vi "Take and analyse picture.vi"(0 "Training image on/off":bool, 1 "8 Insects or less":bool, 2 "Session Out in":T3, 3 "Refnum in":T1, 5 "error in (no error)":errorcluster, 6 "Sample ID":string, 8 "Safe pictures":bool) -> (9 "error out":errorcluster, 10 "output cluster":T2, 14 "Insect-data-array (out of range removed)":dbl[][](array[numeric]), 16 "Number of objects":i32, 17 "Session Out out":T3, 18 "Tegne cirkel array":dbl[][](array[numeric]), 19 "Black image error":bool)   [LabVIEW 2024]
doc: "Collects an image and runs it throu the vision asistent. Then transforms output data to sutible outlets and formats."
uses:
  <vilib>/userDefined/High Color/IMAQdx.ctl
  <vilib>/vision/Image Controls.llb/IMAQ Image.ctl
  <vilib>/vision/NI_Vision_Development_Module.lvlib
  <vilib>/vision/driver/NI_Vision_Acquisition_Software.lvlib
panel:
  out "Camera feed":T1(plugin-control)
  in  "Boolean":bool
  out "Image from vision assistant 2":T1(plugin-control)
  out "T_and_A Stoped":bool
  out "Match Score (Color Matching 1)":i32[](array[numeric])
  out "Objects after sorting":string[][](array[string])
  out "Image from vision assistant":T1(plugin-control)
  in  "Stop program":bool
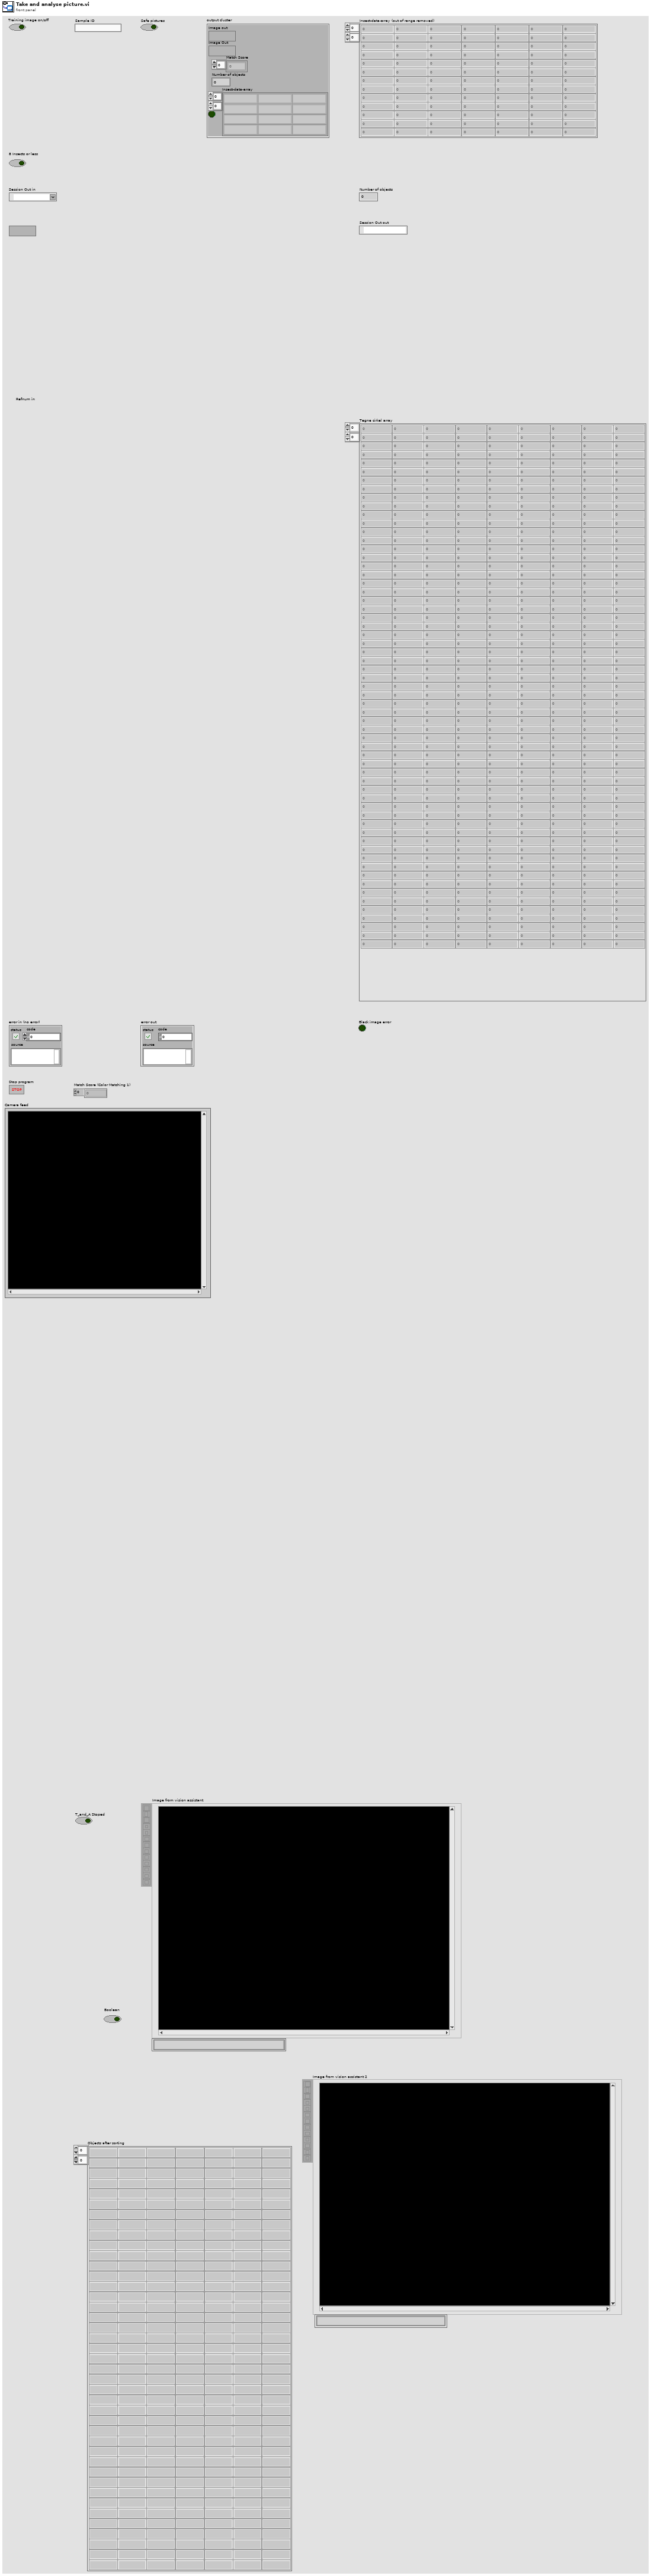
[diagram p1: front panel]
types:
  T1 = typedef "IMAQ Image.ctl" = refnum<image>
  T2 = cluster{"Image out":T1, "Image Out":T1, "Match Score":i32[], "Number of objects":i32, "Insect-data-array":string[][], bool}
  T3 = typedef "IMAQdx.ctl" = refnum<k21>
  T4 = cluster{"Measurement Parameter":i32, "Range Lower Value":dbl, "Range Upper Value":dbl, "Range":bool, "Measurement Type":bool}[]
  T5 = cluster{"Image out":T1, "Image Out":T1, "Match Score (Color Matching 1)":i32[], "Number of objects":i32, "Insect-data-array":string[][], bool}
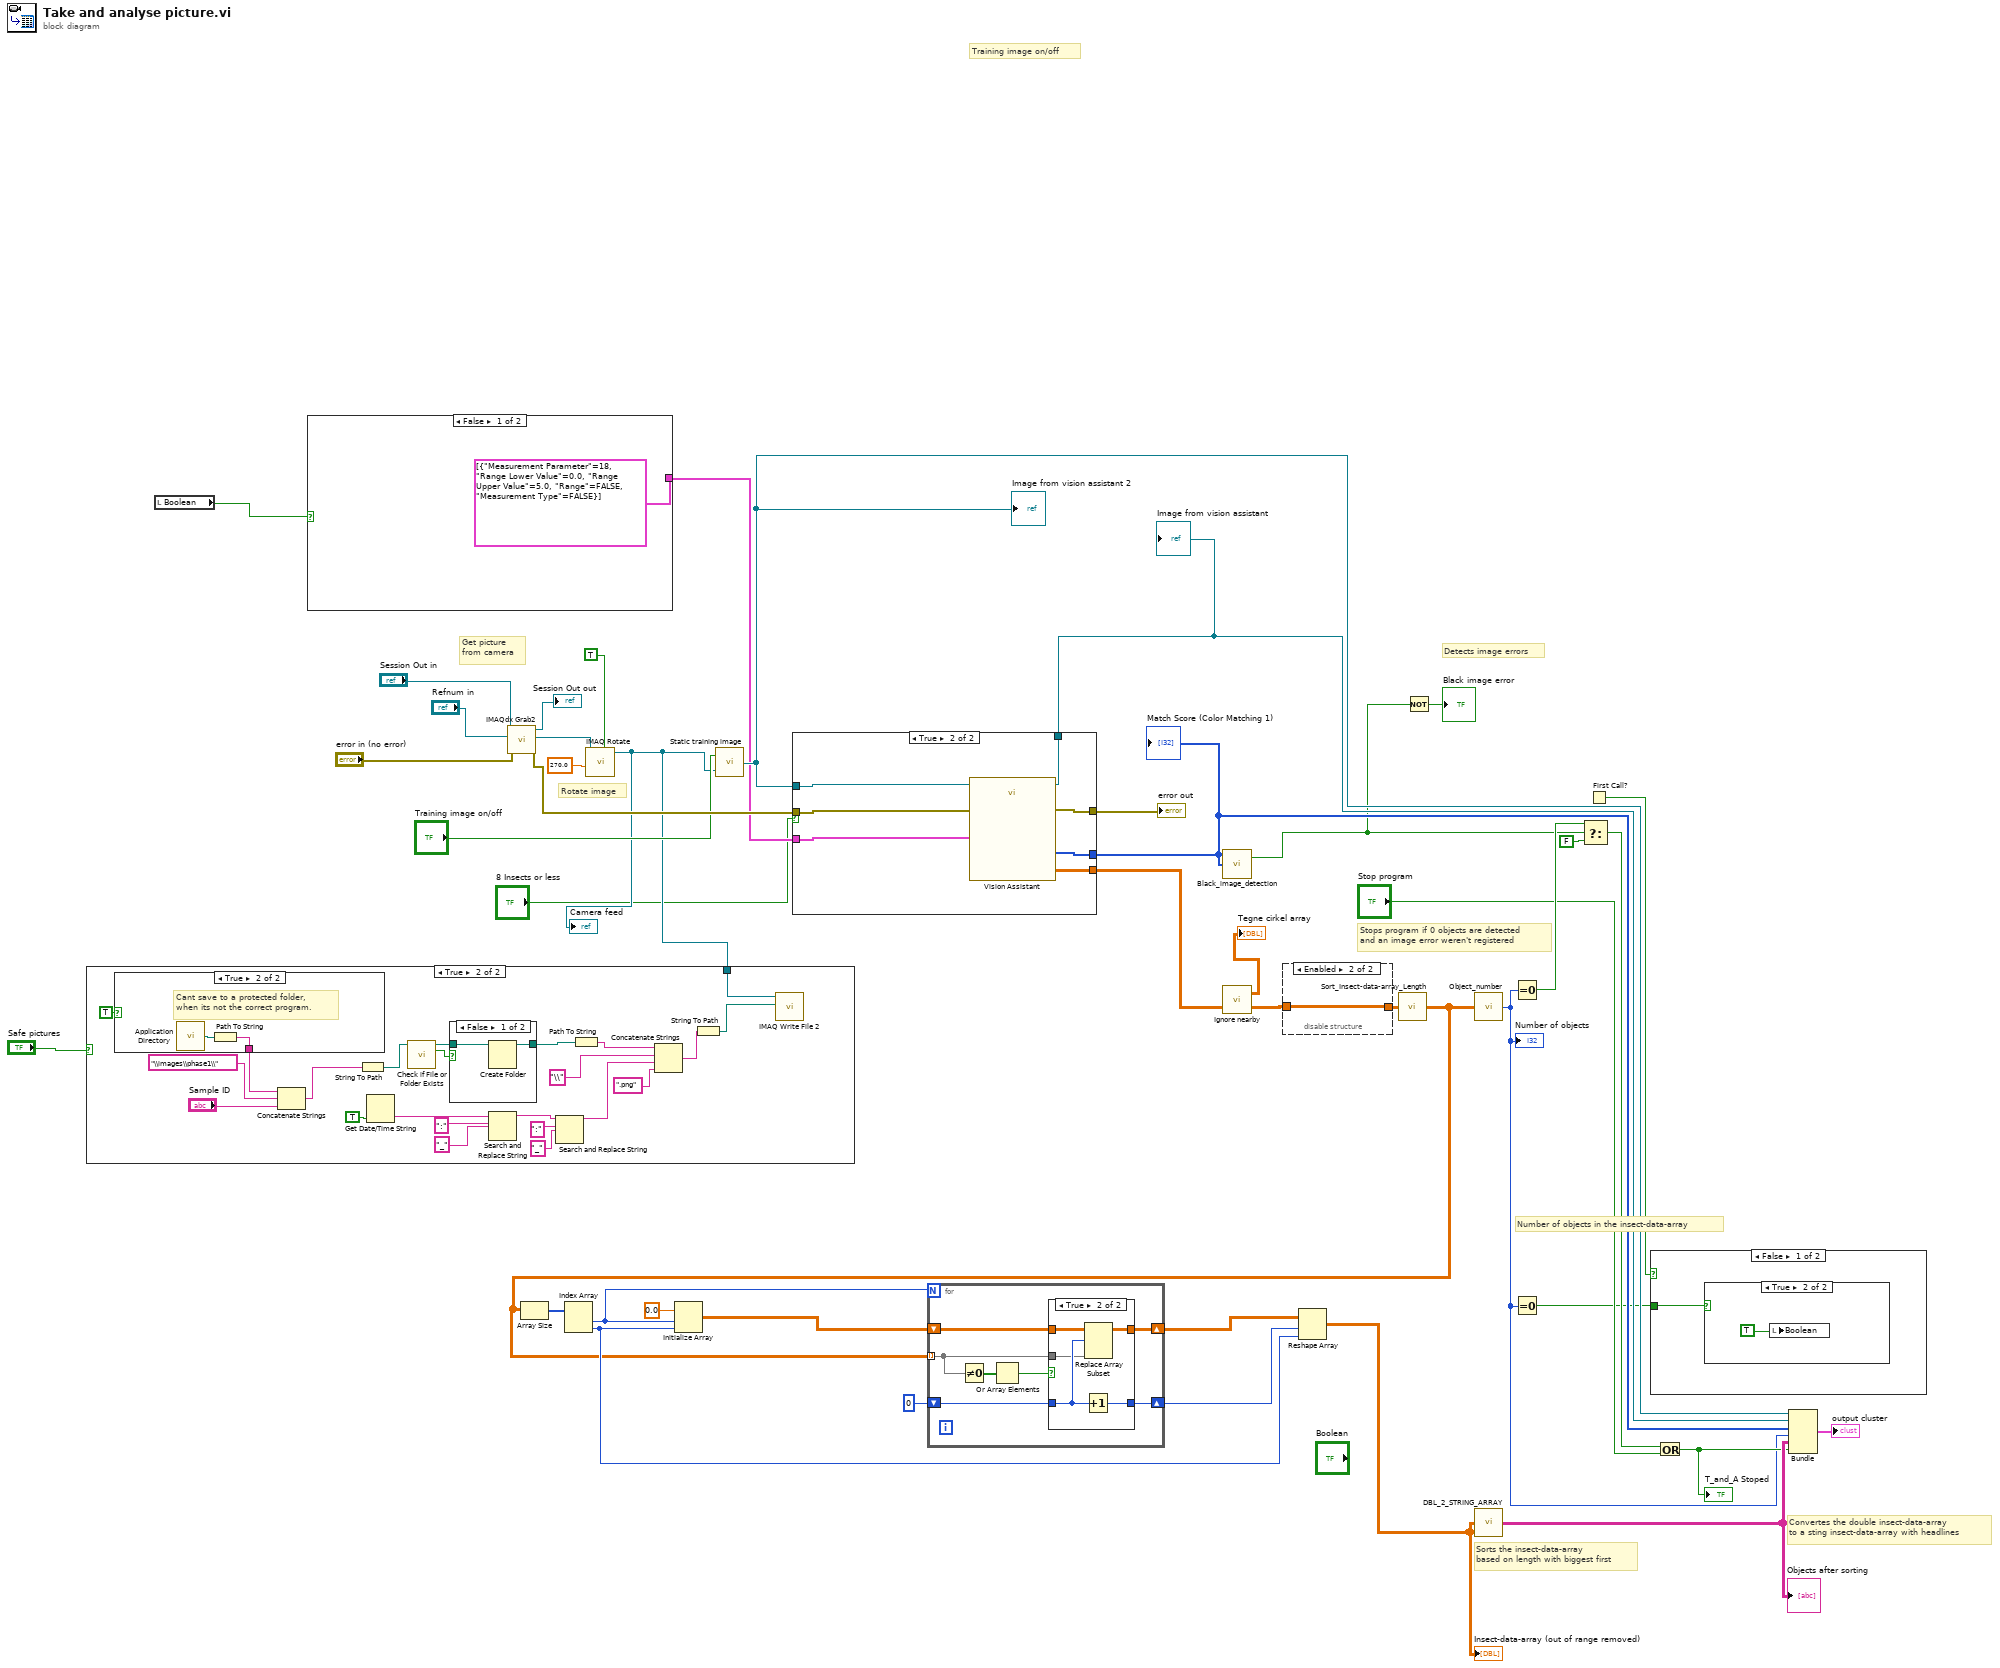
[diagram p0: block diagram]
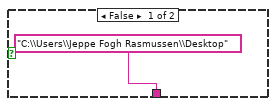
[diagram p3: hidden frame]
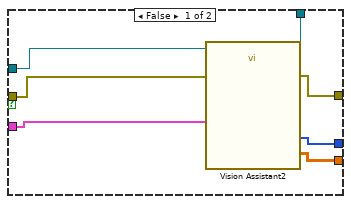
[diagram p5: hidden frame]
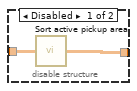
[diagram p6: hidden frame]
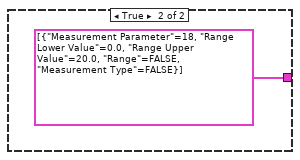
[diagram p8: hidden frame]
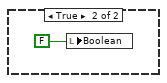
[diagram p10: hidden frame]
diagram:
  # "Detects image errors"
  # "Stops program if 0 objects are detected \nand an image error weren't registered"
  # "Number of objects in the insect-data-array"
  # "Convertes the double insect-data-array\nto a sting insect-data-array with headlines"
  # "Get picture \nfrom camera"
  # "Rotate image"
  # "Training image on/off"
  # "Sorts the insect-data-array\nbased on length with biggest first"
  n1 = local read "Boolean"() -> (w22:bool)
  n2 = case shown="False" w22 {
    tunnel: [T4 [{"Measurement Parameter"=18, "Range Lower Value"=0.0, "Range Upper Value"=5.0, "Range"=FALSE, "Measurement Type"=FALSE}] ("Selection Values (Particle Filter 2)") T4 [{"Measurement Parameter"=18, "Range Lower Value"=0.0, "Range Upper Value"=20.0, "Range"=FALSE, "Measurement Type"=FALSE}] ("Selection Values (Particle Filter 2)")] -> w24
    frame False {
    }
    frame True {
    }
  }
  n3 = call <vilib>:"IMAQdx Grab2.vi"("error in"="error in (no error)", "Image In"="Refnum in", "Session In"="Session Out in") -> ("error out"=w34:errorcluster, "Image Out"=w40:T1, "Session Out"=→"Session Out out":T3)  [unwired: 5 in, 1 out]
  n4 = call "IMAQ Rotate"("Maintain Size"=TRUE, "Angle (degrees)"=sgl 270.0, "Image Src"=w40) -> ("Image Dst Out"=w5:T1)  [unwired: 7 in, 1 out]
  "Camera feed" <- w5
  n5 = case shown="True" "Safe pictures" {
    tunnel: w5 -> [_ w69]
    frame False {
    }
    frame True {
      n6 = case shown="True" TRUE {
        tunnel: ["C:\\Users\\Jeppe Fogh Rasmussen\\Desktop" w72] -> w59
        frame False {
        }
        frame True {
          # "Cant save to a protected folder,\nwhen its not the correct program."
          n7 = call <vilib>:"Application Directory.vi"() -> ("Application Directory"=w71:path)
          n8 = Path To String(path=w71) -> (string=w72:string)
        }
      }
      n9 = Concatenate Strings(w59, "\\images\\phase1\\" ("string"), "Sample ID") -> (w65:string)
      n10 = String To Path(string=w65) -> (path=w64:path)
      n11 = Get Date/Time String(want seconds? (F)=TRUE) -> (time string=w53:string)  [unwired: 2 in, 1 out]
      n12 = call <vilib>:"Check if File or Folder Exists.vi"("path"=w64) -> ("file or folder exists?"=w63:bool, "dup path"=w62:path)  [unwired: 8 in, 1 out]
      n13 = case shown="False" w63 {
        tunnel: w62 -> [w74 w75]
        tunnel: [w73 w75] -> w66
        frame False {
          n14 = Create Folder(path (use dialog)=w74) -> (created path=w73:path)  [unwired: 2 in, 2 out]
        }
        frame True {
        }
      }
      n15 = Search and Replace String(input string=w53, search string=":", replace string="_" ("replace string (\"\")")) -> (result string=w48:string)  [unwired: 5 in, 3 out]
      n16 = Search and Replace String(input string=w48, search string=":", replace string="_" ("replace string (\"\")")) -> (result string=w47:string)  [unwired: 5 in, 3 out]
      n17 = Path To String(path=w66) -> (string=w56:string)
      n18 = Concatenate Strings(w56, "\\" ("string"), w47, ".png" ("string")) -> (w68:string)
      n19 = String To Path(string=w68) -> (path=w67:path)
      n20 = call-poly "IMAQ Write File 2"("File Path"=w67, "Image"=w69) -> ()  [unwired: 8 in, 2 out]
    }
  }
  n21 = call "Static training image.vi"("Image in"=w5, "Training image on/off"="Training image on/off") -> ("Image out"=w35:T1)
  "Image from vision assistant 2" <- w35
  n22 = case shown="True" "8 Insects or less" {
    tunnel: w35 -> [w80 w89]
    tunnel: w34 -> [w81 w88]
    tunnel: [w79 w87] -> w33
    tunnel: [w77 w86] -> w32
    tunnel: [w78 w85] -> w31
    tunnel: [w76 w84] -> w29
    tunnel: w24 -> [w82 w83]
    frame False {
      n23 = call "Vision Assistant2"("Image In"=w80, "Selection Values (Particle Filter 2 Remove small)"=w82, "error in"=w81) -> ("Image Out"=w79:T1, "Particle Measurements (Real-World) (Particle Analysis 1)"=w76:dbl[][], "Match Score (Color Matching 1)"=w77:i32[], "error out"=w78:errorcluster)  [unwired: 21 in]
    }
    frame True {
      n24 = call "Vision Assistant"("Image In"=w89, "Selection Values (Particle Filter 2 Remove small)"=w83, "error in"=w88) -> ("Image Out"=w87:T1, "Particle Measurements (Real-World) (Particle Analysis 1)"=w84:dbl[][], "Match Score (Color Matching 1)"=w86:i32[], "error out"=w85:errorcluster)  [unwired: 21 in]
    }
  }
  "Image from vision assistant" <- w33
  "Match Score (Color Matching 1)" <- w32
  "error out" <- w31
  n25 = call "Black_image_detection.vi"("Match score"=w32) -> ("No Error"=w2:bool)  [unwired: 1 in]
  n26 = call "Ignore nearby.vi"("Particle Measurements (Real-World) (Particle Analysis 1)"=w29) -> ("s? t:f"=w25:dbl[][], "appended array"=→"Tegne cirkel array":dbl[][])  [unwired: 1 in]
  n27 = disable-structure shown="Enabled" {
    disable-tunnel: [w91 w92] -> w30
    disable-tunnel: w25 -> [w90 w92]
    frame Disabled {
      n28 = call "Sort active pickup area.vi"("Insect-data-array"=w90) -> ("Insect-data-array (out of range removed)"=w91:dbl[][])  [unwired: 2 in]
    }
    frame Enabled {
    }
  }
  n29 = call "Sort_Insect-data-array_Length.vi"("Insect-data-array"=w30) -> ("Insect-data-array (sorted-length)"=w9:dbl[][])
  n30 = Array Size(array=w9) -> (size(s)=w16:i32[])
  n31 = Index Array(array=w16) -> (element #1=w14:i32, element #2=w10:i32)  [unwired: 2 in]
  n32 = Initialize Array(0.0, w14, w10) -> (w15:dbl[][])
  n33 = for {
    N: w14 -> [_]
    shift-right: [w99] -> w11
    shift-left: w15 -> [w98]
    shift-right: [w96] -> w12
    shift-left: 0 -> [w97]
    tunnel: w9 -> [w93] mode=indexing
    n34 = Not Equal To 0?(x=w93) -> (x != 0?=w95:bool[])
    n35 = Or Array Elements(Boolean array=w95) -> (logical OR=w94:bool)
    n36 = case shown="True" w94 {
      tunnel: w98 -> [w101 w106]
      tunnel: [w101 w105] -> w99
      tunnel: w97 -> [w100 w103]
      tunnel: [w100 w104] -> w96
      tunnel: w93 -> [_ w102]
      frame False {
      }
      frame True {
        n37 = Increment(x=w103) -> (x+1=w104:i32)
        n38 = Replace Array Subset(array=w106, new element=w102, index (row)=w103) -> (w105:dbl[][])  [unwired: 1 in]
      }
    }
  }
  n39 = Reshape Array(w11, w12, w10) -> (w8:dbl[][])
  "Insect-data-array (out of range removed)" <- w8
  n40 = Not(x=w2) -> (.not. x?=→"Black image error":bool)
  n41 = call "Object_number.vi"("Insect-data-array"=w9) -> ("Number of objects"=w23:i32)
  "Number of objects" <- w23
  n42 = call "DBL_2_STRING_ARRAY.vi"("Insect-data-array"=w8) -> ("Insect-data-array"=w38:string[][])
  "Objects after sorting" <- w38
  n43 = Equal To 0?(x=w23) -> (x = 0?=w42:bool)
  n44 = Equal To 0?(x=w23) -> (x = 0?=w27:bool)
  n45 = Select(t=w42, s=w2, f=FALSE) -> (s? t:f=w43:bool)
  n46 = First Call?() -> (First Call?: T/F=w28:bool)
  n47 = case shown="False" w28 {
    tunnel: w27 -> [w107 _]
    frame False {
      n48 = case shown="True" w107 {
        frame False {
        }
        frame True {
          n49 = local write "Boolean"(TRUE) -> ()
        }
      }
    }
    frame True {
      n50 = local write "Boolean"(FALSE) -> ()
    }
  }
  n51 = Or(x=w43, y="Stop program") -> (x .or. y?=w37:bool)
  "T_and_A Stoped" <- w37
  n52 = Bundle("Image out"=w35, "Image Out"=w33, "Match Score (Color Matching 1)"=w32, "Number of objects"=w23, "Insect-data-array"=w38, w37) -> (→"output cluster":T5)  [unwired: 1 in]
